vi "PotLift.vi"(10 "Pot Position":dbl, 11 "Joystick Y axis":dbl) -> (3 "Scaled Y":dbl)   [LabVIEW 2017]
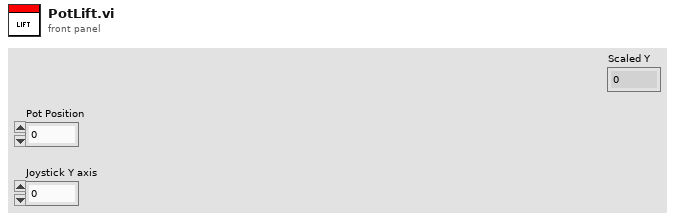
[diagram p1: front panel]
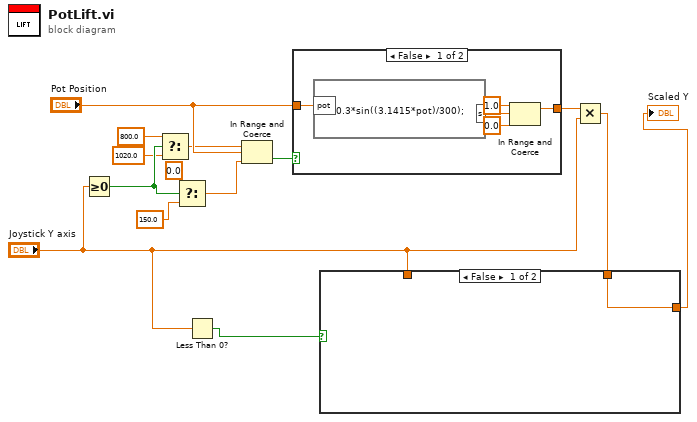
[diagram p0: block diagram]
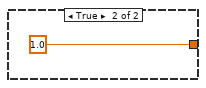
[diagram p3: hidden frame]
diagram:
  n1 = Greater Or Equal To 0?(x="Joystick Y axis") -> (x >= 0?=w11:bool)
  n2 = Select(t=800.0, s=w11, f=1020.0) -> (s? t:f=w8:dbl)
  n3 = Select(t=0.0, s=w11, f=150.0) -> (s? t:f=w7:dbl)
  n4 = Less Than 0?(x="Joystick Y axis") -> (x < 0?=w4:bool)
  n5 = In Range and Coerce(upper limit=w8, x="Pot Position", lower limit=w7) -> (In Range?=w13:bool)  [unwired: 1 out]
  n6 = case shown="False" w13 {
    tunnel: [w16 1.0] -> w14
    tunnel: "Pot Position" -> [w15 _]
    frame False {
      n7 = formula code="s=0.3*sin((3.1415*pot)/300);"("pot"=w15) -> ("s"=w19:dbl)
      n8 = In Range and Coerce(upper limit=1.0, x=w19, lower limit=0.0) -> (coerced(x)=w16:dbl)  [unwired: 1 out]
    }
    frame True {
    }
  }
  n9 = Multiply(x=w14, y="Joystick Y axis") -> (x*y=w1:dbl)
  n10 = case shown="False" w4 {
    tunnel: [w21 w22] -> w2
    tunnel: "Joystick Y axis" -> [_ w22]
    tunnel: w1 -> [w21 _]
    frame False {
    }
    frame True {
    }
  }
  "Scaled Y" <- w2
